vi "Conv1D_LabVIEW.vi"(6 "Kernel Relative Size":sgl=0.001, 7 "No. of Repetition":i32, 11 "Size":i32) -> (3 "Results(s)":dbl format="%.6f")   [LabVIEW 2020]
uses:
  <vilib>/Analysis/NI_AALBase.lvlib
  4e24d26d-fcbb-44a5-9aa8-75639d06e416.vi
  2ed5783d-9886-4979-abaf-b24675aa47c9.vi
  <vilib>/Analysis/NI_AALPro.lvlib
  <vilib>/Analysis/2dsp.llb/1D Convolution (DBL).vi
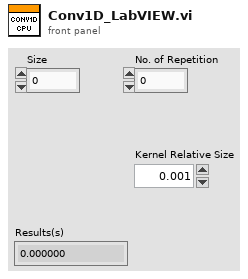
[diagram p1: front panel]
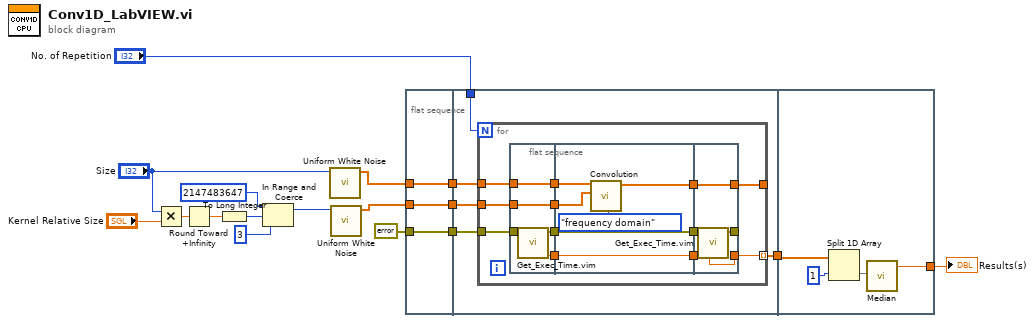
[diagram p0: block diagram]
diagram:
  n1 = Multiply(x="Size", y="Kernel Relative Size") -> (x*y=w13:sgl)
  n2 = Round Toward +Infinity(x=w13) -> (ceil(x): smallest int >= x=w12:sgl)
  n3 = To Long Integer(number=w12) -> (32bit integer=w11:i32)
  n4 = In Range and Coerce(upper limit=2147483647 ("lower limit"), x=w11, lower limit=3) -> (coerced(x)=w15:i32)  [unwired: 1 out]
  n5 = call <vilib>:"Uniform White Noise.vi"("samples"="Size") -> ("uniform white noise"=w4:dbl[])  [unwired: 9 in, 1 out]
  n6 = call <vilib>:"Uniform White Noise.vi"("samples"=w15) -> ("uniform white noise"=w3:dbl[])  [unwired: 9 in, 1 out]
  n7 = flat-sequence {
    tunnel: errorcluster {"status"=FALSE, "code"=0, "source"=""} ("error out") -> [w19]
    tunnel: w4 -> [w20]
    tunnel: [w20] -> w8
    tunnel: [w19] -> w7
    tunnel: w3 -> [w18]
    tunnel: [w18] -> w6
    tunnel: w8 -> [w25]
    tunnel: w7 -> [w24]
    tunnel: [w23] -> w5
    tunnel: w6 -> [w22]
    tunnel: "No. of Repetition" -> [w21]
    tunnel: [w54] -> w1
    tunnel: w5 -> [w57]
    frame #0 {
    }
    frame #1 {
      n8 = for {
        N: w21 -> [_]
        tunnel: w25 -> [w37]
        tunnel: w24 -> [w36]
        tunnel: [w29] -> w23 mode=indexing
        tunnel: w22 -> [w28]
        tunnel: [w26] -> _
        n9 = flat-sequence {
          tunnel: w36 -> [w41]
          tunnel: w37 -> [w42]
          tunnel: [w42] -> w35
          tunnel: [w40] -> w34
          tunnel: [w39] -> w30
          tunnel: w28 -> [w38]
          tunnel: [w38] -> w27
          tunnel: w35 -> [w48]
          tunnel: w34 -> [w46]
          tunnel: [w47] -> w33
          tunnel: [w46] -> w32
          tunnel: [w45] -> w31
          tunnel: w30 -> [w45]
          tunnel: w27 -> [w44]
          tunnel: [w51] -> _
          tunnel: [w53] -> w26
          tunnel: w33 -> [w53]
          tunnel: w32 -> [w52]
          tunnel: w31 -> [w50]
          tunnel: [w49] -> w29
          frame #0 {
            n10 = call "Get_Exec_Time.vim"("error in (no error)"=w41) -> ("T(n)"=w39:dbl, "error out"=w40:errorcluster)  [unwired: 6 in, 1 out]
          }
          frame #1 {
            n11 = call-poly <vilib>:"Convolution.vi"("algorithm"=enum32{"direct", "frequency domain"}."frequency domain", "Y"=w44, "X"=w48) -> ("X * Y"=w47:dbl[])  [unwired: 7 in, 1 out]
          }
          frame #2 {
            n12 = call "Get_Exec_Time.vim"("T(n-1)"=w50, "error in (no error)"=w52) -> ("error out"=w51:errorcluster, "dT"=w49:dbl)  [unwired: 5 in, 1 out]
          }
        }
      }
    }
    frame #2 {
      n13 = Split 1D Array(array=w57, index=1) -> (second subarray=w55:dbl[])  [unwired: 1 out]
      n14 = call <vilib>:"Median.vi"("X"=w55) -> ("median"=w54:dbl)  [unwired: 1 out]
    }
  }
  "Results(s)" <- w1
